vi "LJLogM build log header string.vi"(1 "Names":string[](array[string]), 2 "# Channels":i32, 3 "Start Timestamp":timestamp) -> (0 "Header String":string)   [LabVIEW 2026]
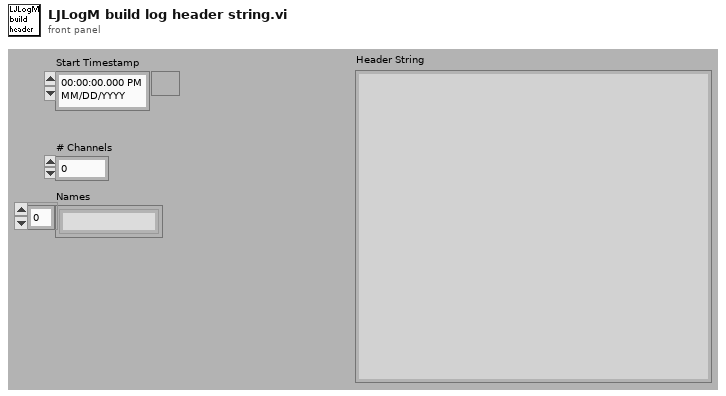
[diagram p1: front panel]
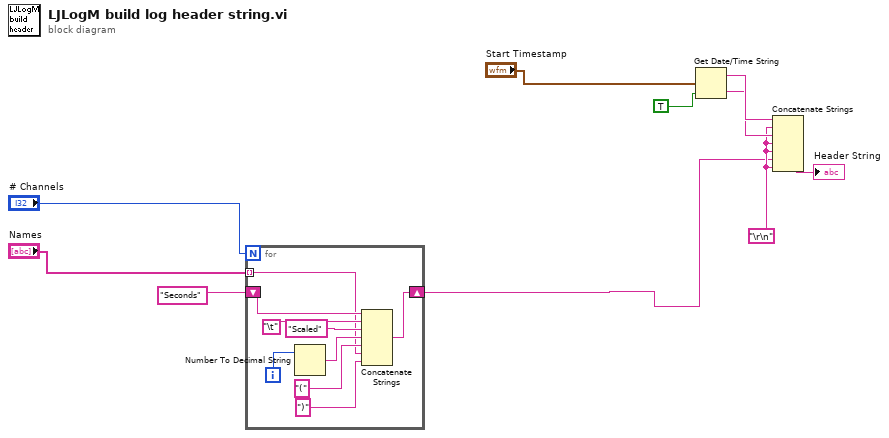
[diagram p0: block diagram]
diagram:
  w6 = "\r\n"
  n1 = for {
    N: "# Channels" -> [_]
    shift-right: [w18] -> w1
    shift-left: "Seconds" ("Substring") -> [w19]
    tunnel: "Names" -> [w12] mode=indexing
    i -> [w16]
    n2 = Number To Decimal String(number=w16) -> (decimal integer string=w15:string)  [unwired: 1 in]
    n3 = Concatenate Strings(w19, "\t", "Scaled" ("string"), w15, "(" ("string"), w12, ")" ("Substring")) -> (w18:string)
  }
  n4 = Get Date/Time String(seconds (now)="Start Timestamp", want seconds? (F)=TRUE) -> (date string=w10:string, time string=w9:string)  [unwired: 1 in]
  n5 = Concatenate Strings(w10, w6, w9, w6, w6, w1, w6) -> (→"Header String":string)
